vi "Store Effect Plugins.vi"(11 "Effects":refnum<class "Effect Interface.lvclass">[](array[class])) -> (3 "Effect Plugin Map":variant)   [LabVIEW 2019, in "Effect Unit.lvclass"]
uses:
  Effect Unit.lvclass
  Plugin Interfaces/Effect Interface/Effect Interface.lvlibp/Plugin Interfaces/Effect Interface/Effect Interface Class/Effect Interface.lvclass
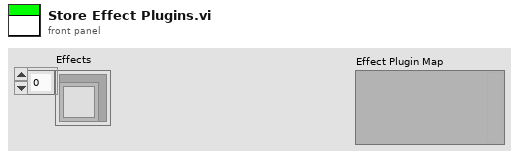
[diagram p1: front panel]
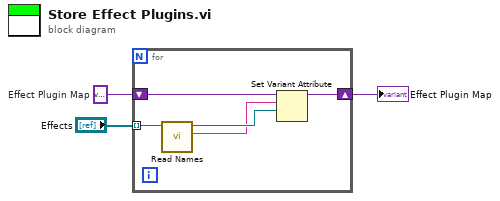
[diagram p0: block diagram]
diagram:
  w2 = variant  # Effect Plugin Map
  n1 = for {
    tunnel: "Effects" -> [w8] mode=indexing
    shift-right: [w5] -> w1
    shift-left: w2 -> [w7]
    n2 = call "Read Names.vi"("Effect Interface in"=w8) -> ("Effect Name"=w4:string, "Effect Interface out"=w6:refnum<class "Effect Interface.lvclass">)  [unwired: 7 in, 2 out]
    n3 = Set Variant Attribute(Variant=w7, name=w4, value=w6) -> (Variant out=w5:variant)  [unwired: 1 in, 2 out]
  }
  "Effect Plugin Map" <- w1
